vi "test Init Value_1.vi"(11 "Test Case In":refnum<class "test EDS.lvclass">) -> (0 "error out":errorcluster, 3 "Test Case Out":refnum<class "test EDS.lvclass">)   [LabVIEW 2024, in "test EDS.lvclass"]
uses:
  test EDS.lvclass
  C:/Program Files/National Instruments/LabVIEW 2024/vi.lib/Astemes/LUnit/Test Case.lvclass
  <vilib>/Astemes/LUnit/Test Case.lvclass/Test Case.ctl
  <vilib>/Astemes/LUnit/Append Fail Result.vi
  <vilib>/Astemes/LUnit/Append Pass Result.vi
  <vilib>/Astemes/LUnit/Run In UI.vi
  <vilib>/Utility/error.llb/Clear Errors.vi
  <vilib>/Astemes/LUnit/Test Case.lvclass
  Core/Value/Value.lvclass
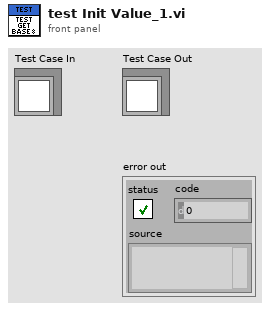
[diagram p1: front panel]
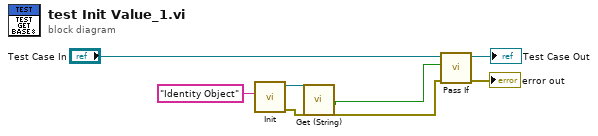
[diagram p0: block diagram]
diagram:
  n1 = call "Init.vi"("Value"="Identity Object") -> ("error out"=w2:errorcluster, "Value out"=w3:refnum<class "Value.lvclass">)  [unwired: 9 in]
  n2 = call "Get (String).vi"("Value in"=w3) -> ("Defined?"=w1:bool)  [unwired: 8 in, 2 out]
  n3 = call <vilib>:"Pass If.vi"("error in (no error)"=w2, "Pass?"=w1, "LUnit Test Case In"="Test Case In") -> ("error out"=→"error out":errorcluster, "LUnit Test Case Out"=→"Test Case Out":refnum<class "test EDS.lvclass">)  [unwired: 7 in]
